vi "Comparador2.vi"() -> ()   [LabVIEW 2019]
uses:
  <vilib>/Native 3D Graph/xcontrol/3DPC_SurfacePlot.xctl
  <vilib>/Utility/file.llb/Read Delimited Spreadsheet (DBL).vi
panel:
  out "3D Graph 2":refnum<class "Base Datatype.lvclass">[](xcontrol)
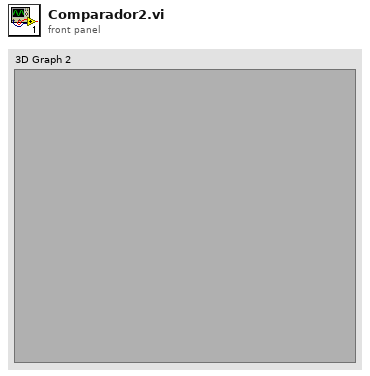
[diagram p1: front panel]
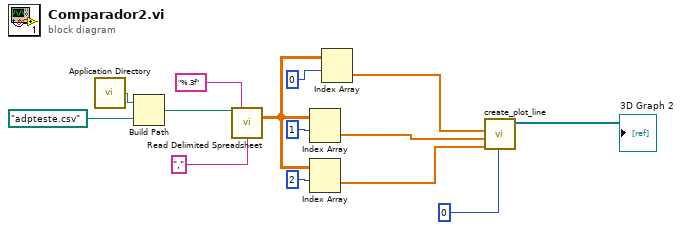
[diagram p0: block diagram]
diagram:
  n1 = call <vilib>:"Application Directory.vi"() -> ("Application Directory"=w12:path)
  n2 = Build Path(base path=w12, name or relative path=path "adpteste.csv" ("file path (dialog if empty)")) -> (appended path=w13:path)
  n3 = call-poly <vilib>:"Read Delimited Spreadsheet.vi"("file path (dialog if empty)"=w13, "format (%.3f)"="%.3f", "delimiter (\\t)"="," ("delimiter (\\t)")) -> ("all rows"=w6:dbl[][])  [unwired: 7 in, 5 out]
  n4 = Index Array(array=w6, index (row)=1) -> (element=w4:dbl[])  [unwired: 1 in]
  n5 = Index Array(array=w6, index (row)=2) -> (element=w3:dbl[])  [unwired: 1 in]
  n6 = Index Array(array=w6, index (row)=0) -> (element=w5:dbl[])  [unwired: 1 in]
  n7 = call <vilib>:"create_plot_line.vi"("plot ID"=0, "z vector"=w3, "y vector"=w4, "x vector"=w5) -> ("plots out"=→"3D Graph 2":refnum<class "Base Datatype.lvclass">[])  [unwired: 1 in, 6 out]
